vi "Fast Draw Object Event.vi"(4 "Fast Draw Action":enum16{"Update", "Remove", "Nothing"}(ring), 7 "Multiplot Representation In":T3, 8 "error in (no error)":errorcluster, 9 "Object Cluster In":T6, 10 "Actual Transform In":T1, 11 "3D Plot.lvclass in":refnum<class "3D Plot.lvclass">) -> (0 "error out":errorcluster, 1 "Object Cluster Out":T6, 2 "Actual Transform Out":T1, 3 "3D Plot.lvclass out":refnum<class "3D Plot.lvclass">, 5 "Multiplot Representation Out":T3)   [LabVIEW 2020, in "3D Plot.lvclass"]
uses:
  3D Plot.lvclass
  Object Cluster.ctl
  Multiplot Representation.ctl
  Plot Representation.ctl
  Range Clusters.ctl
  Mesh Data.ctl
  Actual Transform.ctl
  NI_3D Picture Control.lvlib
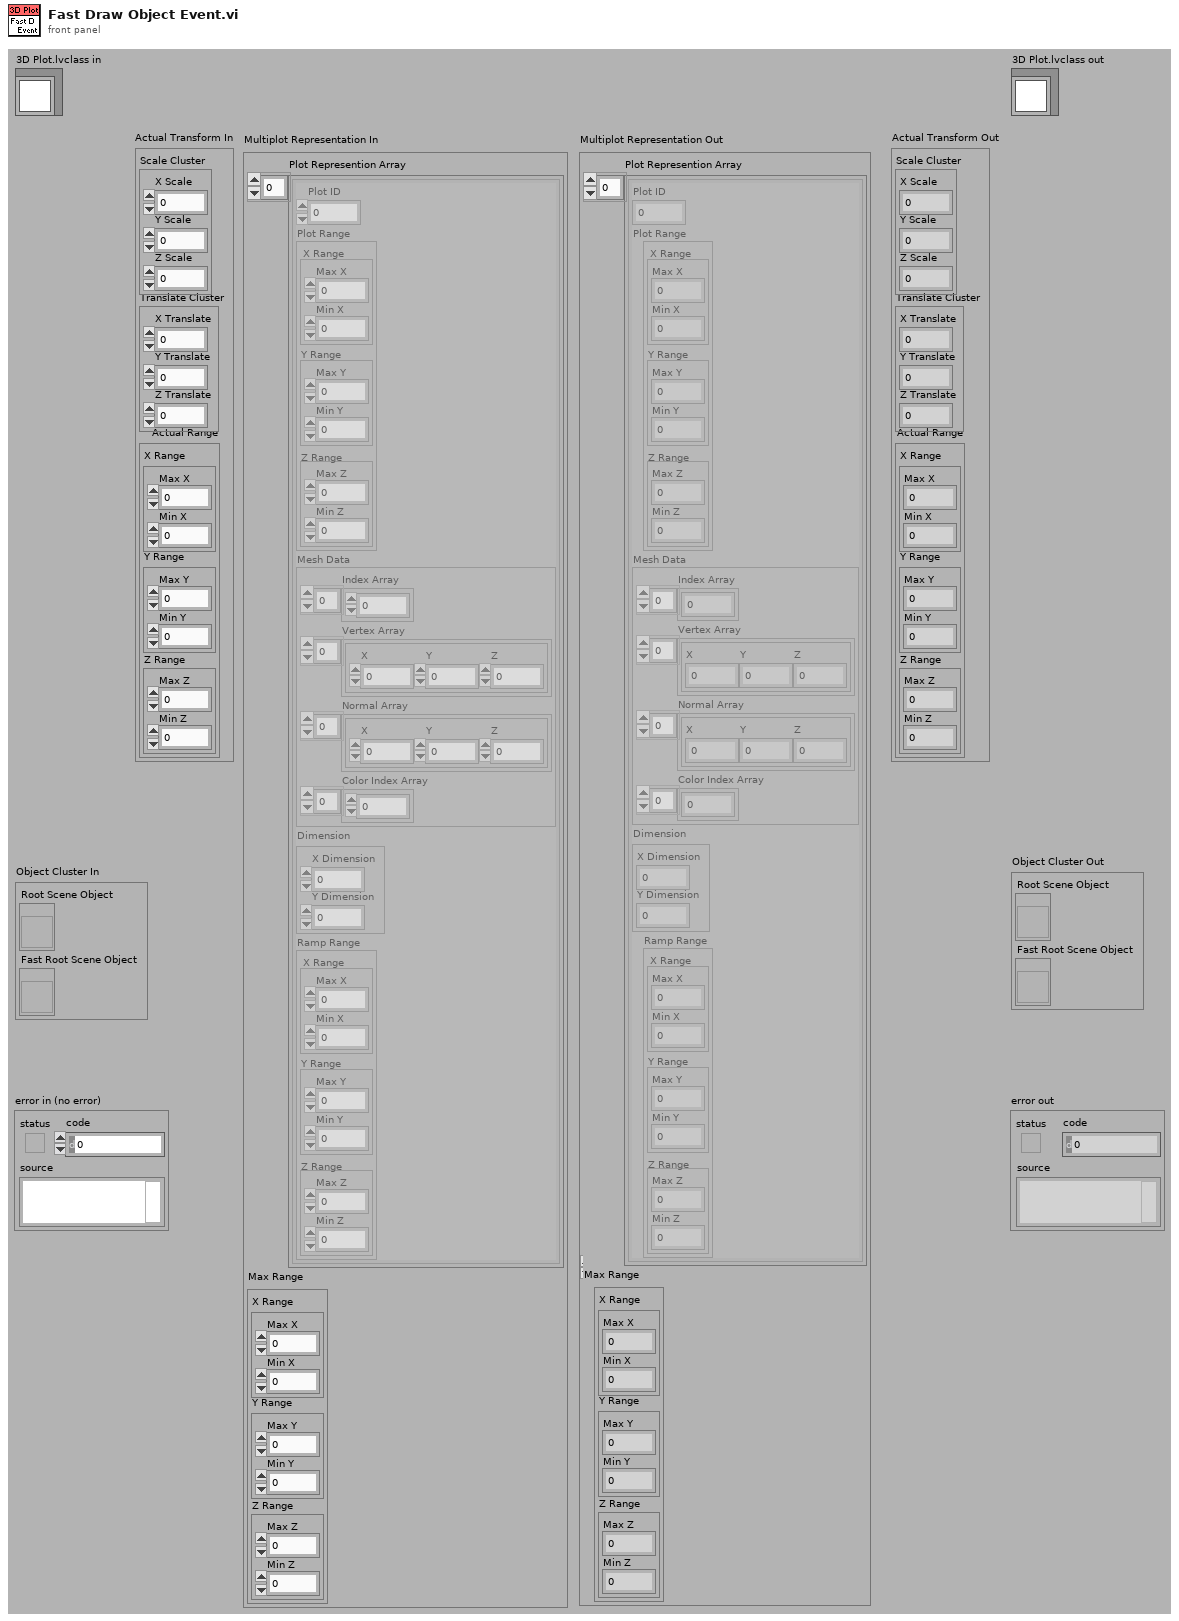
[diagram p1: front panel]
types:
  T1 = typedef "3D Plot.lvclass/Actual Transform.ctl" = cluster{"Scale Cluster":cluster{"X Scale":sgl, "Y Scale":sgl, "Z Scale":sgl}, "Translate Cluster":cluster{"X Translate":sgl, "Y Translate":sgl, "Z Translate":sgl}, "Actual Range":T2}
  T2 = typedef "3D Plot.lvclass/Range Clusters.ctl" = cluster{"X Range":cluster{"Max X":sgl, "Min X":sgl}, "Y Range":cluster{"Max Y":sgl, "Min Y":sgl}, "Z Range":cluster{"Max Z":sgl, "Min Z":sgl}}
  T3 = typedef "3D Plot.lvclass/Multiplot Representation.ctl" = cluster{"Plot Represention Array":T4[], "Max Range":T2}
  T4 = typedef "3D Plot.lvclass/Plot Representation.ctl" = cluster{"Plot ID":i32, "Plot Range":T2, "Mesh Data":T5, "Dimension":cluster{"X Dimension":i32, "Y Dimension":i32}, "Ramp Range":T2}
  T5 = typedef "3D Plot.lvclass/Mesh Data.ctl" = cluster{"Index Array":u32[], "Vertex Array":cluster{"X":sgl, "Y":sgl, "Z":sgl}[], "Normal Array":cluster{"X":sgl, "Y":sgl, "Z":sgl}[], "Color Index Array":i32[]}
  T6 = typedef "3D Plot.lvclass/Object Cluster.ctl" = cluster{"Root Scene Object":refnum<vi>, "Fast Root Scene Object":refnum<vi>}
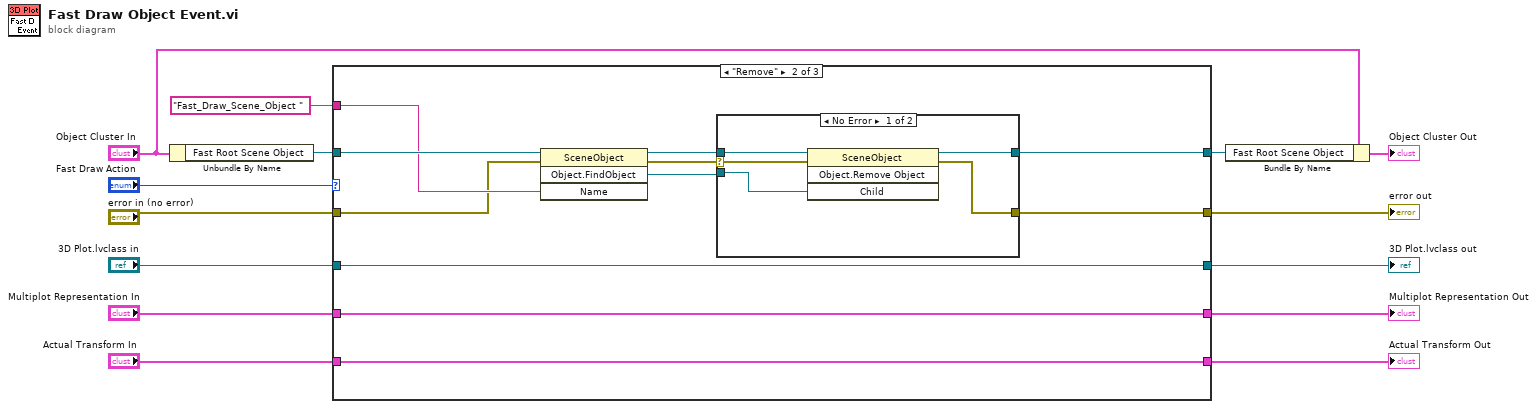
[diagram p0: block diagram]
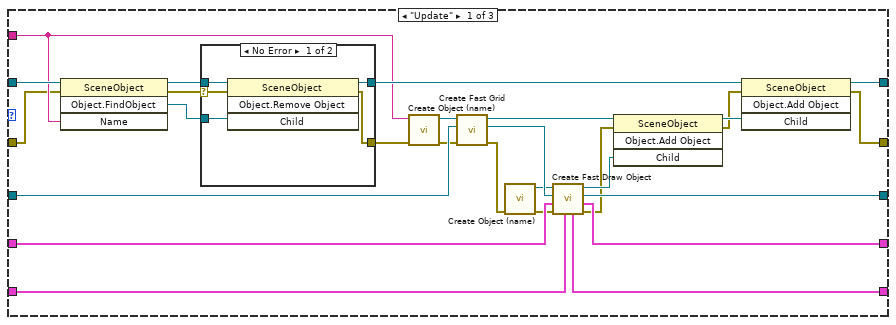
[diagram p2: hidden frame]
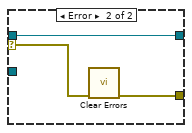
[diagram p3: hidden frame]
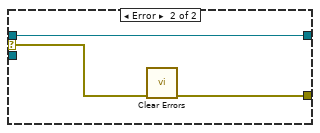
[diagram p4: hidden frame]
diagram:
  n1 = Unbundle By Name("Object Cluster In") -> ("Fast Root Scene Object"=w13:refnum<vi>)
  n2 = case shown="\"Remove\"" "Fast Draw Action" {
    tunnel: [w31 w53 w73] -> w11
    tunnel: w13 -> [w37 w55 w73]
    tunnel: "3D Plot.lvclass in" -> [w28 w60 w71]
    tunnel: "error in (no error)" -> [w16 w51 w72]
    tunnel: [w30 w54 w72] -> w9
    tunnel: [w32 w60 w71] -> w6
    tunnel: [w41 w59 w70] -> w5
    tunnel: "Multiplot Representation In" -> [w40 w59 w70]
    tunnel: "Actual Transform In" -> [w39 w58 w69]
    tunnel: [w38 w58 w69] -> w2
    tunnel: "Fast_Draw_Scene_Object " ("Name") -> [w17 w52 _]
    frame "Update" {
      n3 = invoke class="SceneObject" method="Object.FindObject"(reference=w37, error in=w16, "Name"=w17) -> (reference out=w36:refnum<vi>, error out=w15:errorcluster, "FindObject"=w35:refnum<vi>)  [unwired: 1 in, 1 out]
      n4 = case shown="No Error" w15 {
        selector: w15 -> [w42 w48]
        tunnel: [w44 w47] -> w19
        tunnel: w36 -> [w46 w49]
        tunnel: w35 -> [w45 _]
        tunnel: [w43 w49] -> w34
        frame No Error {
          n5 = invoke class="SceneObject" method="Object.Remove Object"(reference=w46, error in=w42, "Child"=w45) -> (reference out=w43:refnum<vi>, error out=w44:errorcluster)  [unwired: 1 in, 2 out]
        }
        frame Error {
          n6 = call "Clear Errors.vi"("error in (no error)"=w48) -> ("error out"=w47:errorcluster)  [unwired: 5 in, 1 out]
        }
      }
      n7 = call "Create Object (name).vi"("error in (no error)"=w19, "Name"=w17) -> ("error out"=w20:errorcluster, "Scene:New Object"=w29:refnum<vi>)  [unwired: 8 in]
      n8 = call "Create Fast Grid.vi"("error in (no error)"=w20, "3D Plot.lvclass in"=w28, "Fast Draw Object In"=w29) -> ("error out"=w18:errorcluster, "3D Plot.lvclass out"=w27:refnum<class "3D Plot.lvclass">, "Fast Draw Object Out"=w25:refnum<vi>)  [unwired: 6 out]
      n9 = call "Create Object (name).vi"("error in (no error)"=w18) -> ("error out"=w33:errorcluster, "Scene:New Object"=w26:refnum<vi>)  [unwired: 9 in]
      n10 = call-dynamic "Create Fast Draw Object.vi"("Actual Transform In"=w39, "error in (no error)"=w33, "Multiplot Representation In"=w40, "3D Plot.lvclass in"=w27, "Plot Object In"=w26) -> ("error out"=w22:errorcluster, "Multiplot Representation Out"=w41:T3, "3D Plot.lvclass out"=w32:refnum<class "3D Plot.lvclass">, "Plot Object Out"=w24:refnum<vi>, "Actual Transform Out"=w38:T1)  [unwired: 2 out]
      n11 = invoke class="SceneObject" method="Object.Add Object"(reference=w25, error in=w22, "Child"=w24) -> (reference out=w23:refnum<vi>, error out=w21:errorcluster)  [unwired: 1 in, 2 out]
      n12 = invoke class="SceneObject" method="Object.Add Object"(reference=w34, error in=w21, "Child"=w23) -> (reference out=w31:refnum<vi>, error out=w30:errorcluster)  [unwired: 1 in, 2 out]
    }
    frame "Remove" {
      n13 = invoke class="SceneObject" method="Object.FindObject"(reference=w55, error in=w51, "Name"=w52) -> (reference out=w57:refnum<vi>, error out=w50:errorcluster, "FindObject"=w56:refnum<vi>)  [unwired: 1 in, 1 out]
      n14 = case shown="No Error" w50 {
        selector: w50 -> [w61 w67]
        tunnel: [w63 w66] -> w54
        tunnel: w57 -> [w65 w68]
        tunnel: w56 -> [w64 _]
        tunnel: [w62 w68] -> w53
        frame No Error {
          n15 = invoke class="SceneObject" method="Object.Remove Object"(reference=w65, error in=w61, "Child"=w64) -> (reference out=w62:refnum<vi>, error out=w63:errorcluster)  [unwired: 1 in, 2 out]
        }
        frame Error {
          n16 = call "Clear Errors.vi"("error in (no error)"=w67) -> ("error out"=w66:errorcluster)  [unwired: 5 in, 1 out]
        }
      }
    }
    frame "Nothing", Default {
    }
  }
  "error out" <- w9
  "3D Plot.lvclass out" <- w6
  "Multiplot Representation Out" <- w5
  "Actual Transform Out" <- w2
  n17 = Bundle By Name(cluster="Object Cluster In", "Fast Root Scene Object"=w11) -> (→"Object Cluster Out":T6)
